vi "DSF.Engine.Sequencer Bundle.Set Transfer Group Timings.vi"(8 "error in (no error)":errorcluster, 10 "Transfer Group Timings":refnum<class "DSF.Shared.Timing.lvclass">[](array[class]), 11 "Sequencer Bundle in":refnum<class "DSF.Engine.Sequencer.Timing Bundle.lvclass">) -> (0 "error out":errorcluster, 3 "Sequencer Bundle out":refnum<class "DSF.Engine.Sequencer.Timing Bundle.lvclass">)   [LabVIEW 2017, in "DSF.Engine.lvlib" / "DSF.Engine.Sequencer.Timing Bundle.lvclass"]
uses:
  DSF.Engine.Sequencer.Timing Bundle.lvclass
  Shared/Classes/Timing/DSF.Shared.Timing.lvclass
  DSF.Engine.Sequencer.Timing Bundle.lvclass/DSF.Engine.Sequencer.Timing Bundle.ctl
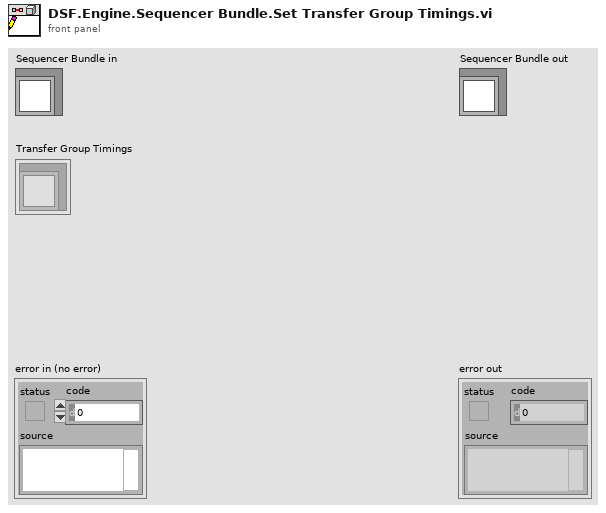
[diagram p1: front panel]
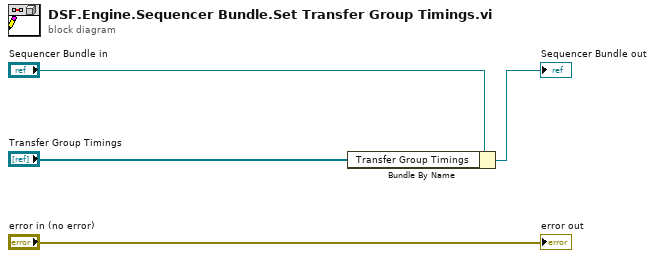
[diagram p0: block diagram]
diagram:
  n1 = Bundle By Name(cluster="Sequencer Bundle in", "Transfer Group Timings"="Transfer Group Timings") -> (→"Sequencer Bundle out":refnum<class "DSF.Engine.Sequencer.Timing Bundle.lvclass">)
  "error out" <- "error in (no error)"
